vi "TimeMode Enum to Boolean.vi"(11 "RelativeTime?":T1) -> (3 "TimeMode":bool)   [LabVIEW 2017, in "GetSetShared.lvlib"]
uses:
  <vilib>/express/express signal manip/GetorSetDDTAttributes/Shared VIs/GetSetShared.lvlib
  <vilib>/express/express signal manip/GetorSetDDTAttributes/Shared VIs/TimeType.ctl
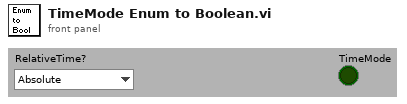
[diagram p1: front panel]
types:
  T1 = typedef "GetSetShared.lvlib/TimeType.ctl" = enum16{"Absolute", "Relative"}
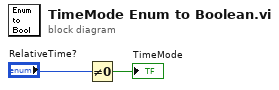
[diagram p0: block diagram]
diagram:
  n1 = Not Equal To 0?(x="RelativeTime?") -> (x != 0?=→"TimeMode":bool)
